vi "CreateLogFile.vi"(8 "error in":errorcluster) -> (0 "error out":errorcluster)   [LabVIEW 2013]
uses:
  Global.vi
  <vilib>/Utility/file.llb/Write To Spreadsheet File (string).vi
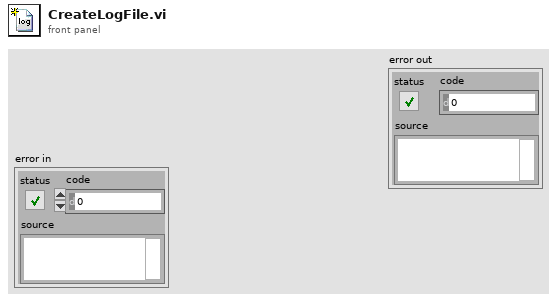
[diagram p1: front panel]
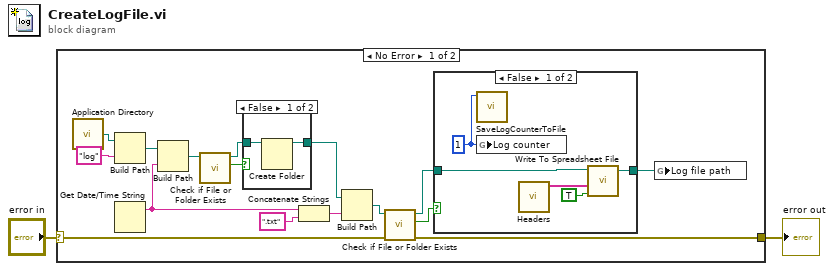
[diagram p0: block diagram]
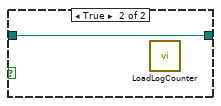
[diagram p3: hidden frame]
diagram:
  n1 = case shown="No Error" "error in" {
    selector: "error in" -> [w14 w28]
    tunnel: [w13 w28] -> w1
    frame No Error {
      n2 = call <vilib>:"Application Directory.vi"() -> ("Application Directory"=w12:path)
      n3 = Build Path(base path=w12, name or relative path="log") -> (appended path=w7:path)
      n4 = Get Date/Time String() -> (date string=w9:string)  [unwired: 3 in, 1 out]
      n5 = Build Path(base path=w7, name or relative path=w9) -> (appended path=w6:path)
      n6 = call <vilib>:"Check if File or Folder Exists.vi"("path"=w6) -> ("file or folder exists?"=w8:bool, "dup path"=w5:path)  [unwired: 8 in, 1 out]
      n7 = case shown="False" w8 {
        tunnel: w5 -> [w20 w21]
        tunnel: [w19 w21] -> w4
        frame False {
          n8 = Create Folder(path (use dialog)=w20) -> (created path=w19:path)  [unwired: 2 in, 2 out]
        }
        frame True {
        }
      }
      n9 = Concatenate Strings(w9, ".txt") -> (w17:string)
      n10 = Build Path(base path=w4, name or relative path=w17) -> (appended path=w3:path)
      n11 = call <vilib>:"Check if File or Folder Exists.vi"("error in (no error)"=w14, "path"=w3) -> ("error out"=w13:errorcluster, "file or folder exists?"=w16:bool, "dup path"=w15:path)  [unwired: 7 in]
      n12 = case shown="False" w16 {
        tunnel: w15 -> [w25 w27]
        tunnel: [w23 w27] -> w10
        frame False {
          w24 = 1 ("Log counter")
          n13 = call "SaveLogCounterToFile.vi"("number"=w24) -> ()  [unwired: 11 in]
          n14 = global write "Global.vi" "Log counter"(w24) -> ()
          n15 = call "Headers.vi"() -> ("Headers"=w22:string[])  [unwired: 11 in]
          n16 = call-poly <vilib>:"Write To Spreadsheet File.vi"("append to file? (new file:F)"=TRUE, "1D data"=w22, "file path (dialog if empty)"=w25) -> ("new file path (Not A Path if cancelled)"=w23:path)  [unwired: 5 in]
        }
        frame True {
          n17 = call "LoadLogCounter.vi"() -> ()  [unwired: 12 in]
        }
      }
      n18 = global write "Global.vi" "Log file path"(w10) -> ()
    }
    frame Error {
    }
  }
  "error out" <- w1
